vi "Init.vi"(0 "Size":u16, 1 "Game Difficulty Out":u32(ring)=750 items=["Easy"=750, "Hard"=500, "Extreme"=300, "Carlo Music"=150], 2 "SCORE":refnum<vi>, 5 "Score":refnum<vi>, 7 "Board Game":refnum<vi>, 9 "Shield":refnum<vi>, 11 "error in (no error)":errorcluster, 12 "Colour":u32(colorbox)) -> (4 "Board Game out":refnum<class "Board Game.lvclass">, 15 "error out":errorcluster)   [LabVIEW 2021, in "Board Game.lvclass"]
uses:
  Board Game.lvclass
  Application/Shield.ctl
  Board Game.lvclass/Board Game.ctl
  Application/Game.lvclass
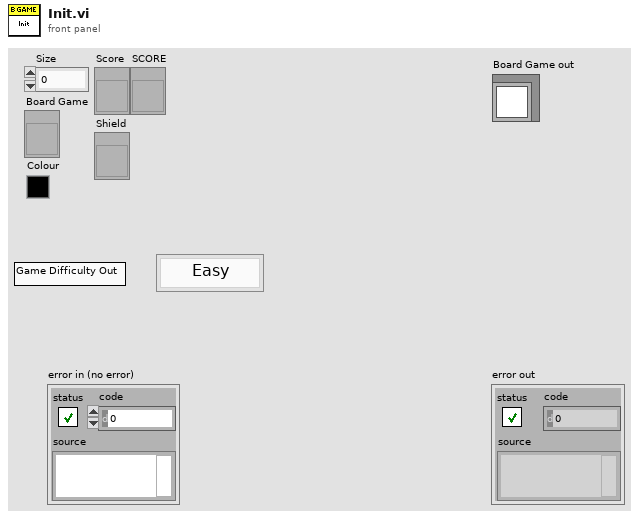
[diagram p1: front panel]
types:
  T1 = enum8{"Enabled", "Disabled", "Disabled and Grayed Out"}
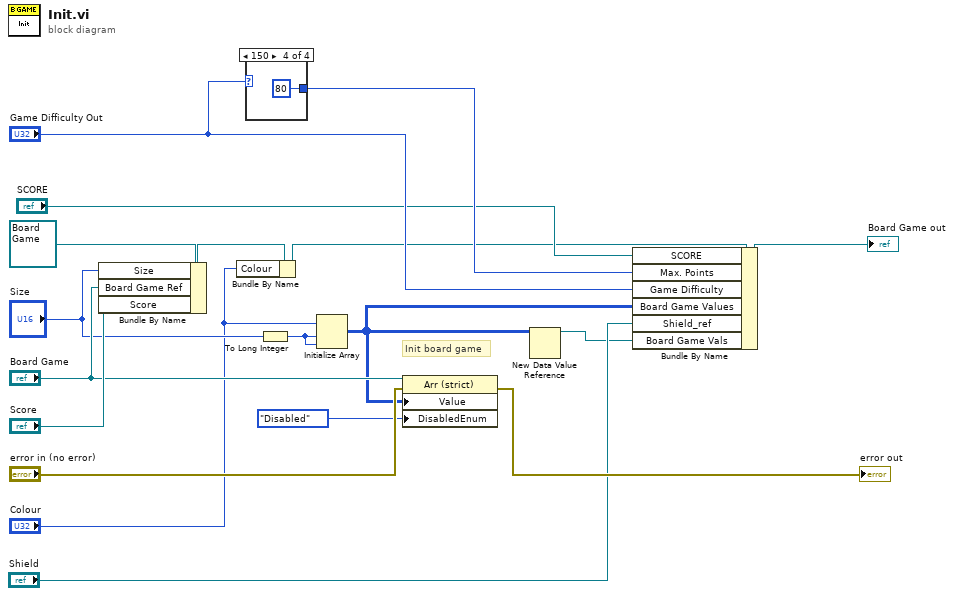
[diagram p0: block diagram]
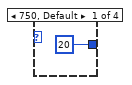
[diagram p2: hidden frame]
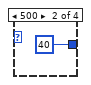
[diagram p3: hidden frame]
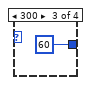
[diagram p4: hidden frame]
diagram:
  # "Init board game"
  n1 = Bundle By Name(cluster=refnum<class "Board Game.lvclass"> refnum ("Board Game out"), "Size"="Size", "Board Game Ref"="Board Game", "Score"="Score") -> (w3:refnum<class "Board Game.lvclass">)
  n2 = Bundle By Name(cluster=w3, "Colour"="Colour") -> (w2:refnum<class "Board Game.lvclass">)
  n3 = case shown="150" "Game Difficulty Out" {
    tunnel: [u16 20 ("Max. Points") u16 40 ("Max. Points") u16 60 ("Max. Points") u16 80 ("Max. Points")] -> w8
    frame 750, Default {
    }
    frame 500 {
    }
    frame 300 {
    }
    frame 150 {
    }
  }
  n4 = To Long Integer(number="Size") -> (32bit integer=w12:i32)
  n5 = Initialize Array("Colour", w12, w12) -> (w5:u32[][])
  n6 = property class="Arr (strict)"(reference="Board Game", error in="error in (no error)", "Value"=w5, "DisabledEnum"=T1."Disabled" ("Disabled")) -> (error out=→"error out":errorcluster)  [unwired: 1 out]
  n7 = New Data Value Reference(data value=w5) -> (data value reference=w4:refnum<data-value>)  [unwired: 1 in, 1 out]
  n8 = Bundle By Name(cluster=w2, "SCORE"="SCORE", "Max. Points"=w8, "Game Difficulty"="Game Difficulty Out", "Board Game Values"=w5, "Shield_ref"="Shield", "Board Game Vals"=w4) -> (→"Board Game out":refnum<class "Board Game.lvclass">)
